vi "Unlock Enclosure Door.vi"(4 "error in":errorcluster, 6 "Unlock Encloure Door":bool) -> (0 "error out":errorcluster)   [LabVIEW 2015]
uses:
  <vilib>/DAQmx/write.llb/DAQmx Write (Digital Bool 1Line 1Point).vi
  <vilib>/DAQmx/miscellaneous.llb/DAQmx Fill In Error Info.vi
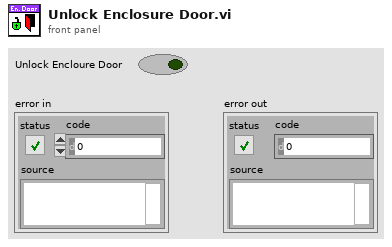
[diagram p1: front panel]
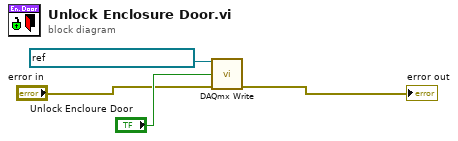
[diagram p0: block diagram]
diagram:
  n1 = call-poly <vilib>:"DAQmx Write.vi"("task/channels in"=refnum<k21> "DO7 Unlock Door Request" ("DAQmx Global Channel"), "data"="Unlock Encloure Door", "error in"="error in") -> ("error out"=→"error out":errorcluster)  [unwired: 10 in, 2 out]
